vi "verify communication.vi"(8 "error in (no error)":errorcluster, 11 "Server in":refnum<class "Server.lvclass">) -> (0 "error out":errorcluster, 3 "Server out":refnum<class "Server.lvclass">)   [LabVIEW 2018, in "Server.lvclass"]
uses:
  Server.lvclass
  Server.lvclass/Server.ctl
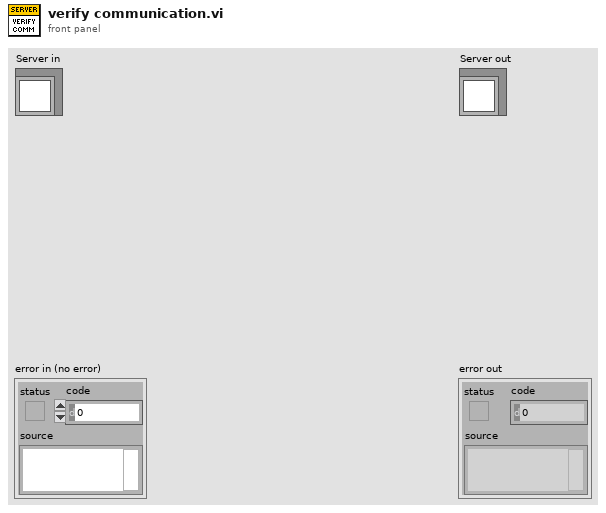
[diagram p1: front panel]
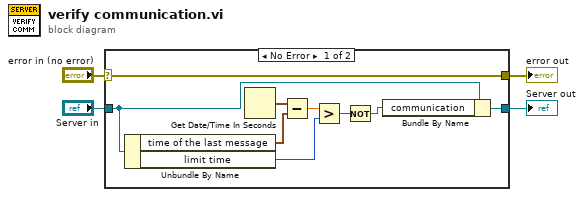
[diagram p0: block diagram]
diagram:
  n1 = case shown="No Error" "error in (no error)" {
    selector: "error in (no error)" -> [w13 w15]
    tunnel: [w13 w15] -> w3
    tunnel: [w7 w14] -> w1
    tunnel: "Server in" -> [w8 w14]
    frame No Error {
      n2 = Unbundle By Name(w8) -> ("time of the last message"=w11:timestamp, "limit time"=w9:u16)
      n3 = Get Date/Time In Seconds() -> (seconds since 1Jan1904=w12:timestamp)
      n4 = Subtract(x=w12, y=w11) -> (x-y=w10:dbl)
      n5 = Greater?(x=w10, y=w9) -> (0:w6:bool)
      n6 = Not(x=w6) -> (.not. x?=w5:bool)
      n7 = Bundle By Name(cluster=w8, "communication"=w5) -> (w7:refnum<class "Server.lvclass">)
    }
    frame Error {
    }
  }
  "error out" <- w3
  "Server out" <- w1
